vi "Multiply.vi"(8 "error in (no error)":errorcluster, 10 "Scale":dbl format="%#_13g", 11 "Field in":refnum<class "Field.lvclass">) -> (0 "error out":errorcluster, 3 "Field out":refnum<class "Field.lvclass">)   [LabVIEW 2020, in "Field.lvclass"]
uses:
  Field.lvclass
  Field.lvclass/Field.ctl
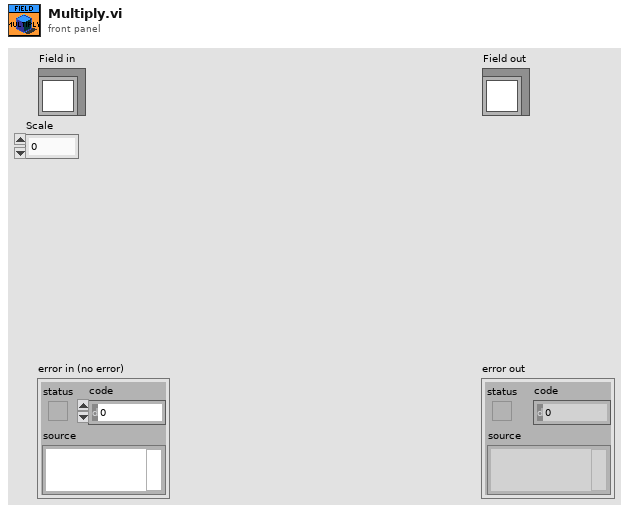
[diagram p1: front panel]
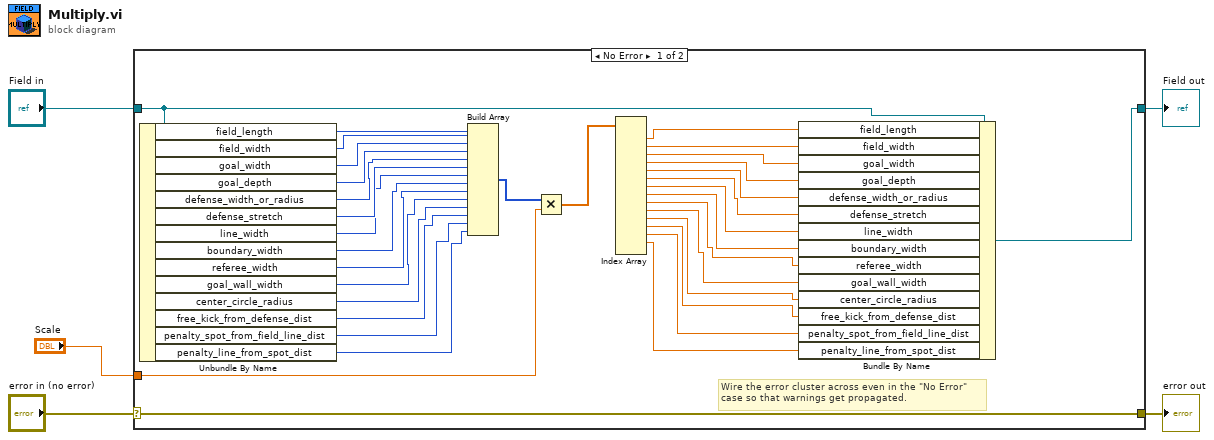
[diagram p0: block diagram]
diagram:
  n1 = case shown="No Error" "error in (no error)" {
    selector: "error in (no error)" -> [w39 w41]
    tunnel: [w39 w41] -> w4
    tunnel: [w37 w40] -> w2
    tunnel: "Field in" -> [w38 w40]
    tunnel: "Scale" -> [w30 _]
    frame No Error {
      # "Wire the error cluster across even in the \"No Error\"\ncase so that warnings get propagated."
      n2 = Unbundle By Name(w38) -> ("field_length"=w36:i32, "field_width"=w35:i32, "goal_width"=w34:i32, "goal_depth"=w33:i32, "defense_width_or_radius"=w32:i32, "defense_stretch"=w31:i32, "line_width"=w14:i32, "boundary_width"=w13:i32, "referee_width"=w12:i32, "goal_wall_width"=w11:i32, "center_circle_radius"=w10:i32, "free_kick_from_defense_dist"=w9:i32, "penalty_spot_from_field_line_dist"=w8:i32, "penalty_line_from_spot_dist"=w7:i32)
      n3 = Build Array(w36, w35, w34, w33, w32, w31, w14, w13, w12, w11, w10, w9, w8, w7) -> (w6:i32[])
      n4 = Multiply(x=w6, y=w30) -> (x*y=w29:dbl[])
      n5 = Index Array(array=w29) -> (element #1=w28:dbl, element #2=w27:dbl, element #3=w26:dbl, element #4=w25:dbl, element #5=w24:dbl, element #6=w23:dbl, element #7=w22:dbl, element #8=w21:dbl, element #9=w20:dbl, element #10=w19:dbl, element #11=w18:dbl, element #12=w17:dbl, element #13=w16:dbl, element #14=w15:dbl)  [unwired: 15 in, 1 out]
      n6 = Bundle By Name(cluster=w38, "field_length"=w28, "field_width"=w27, "goal_width"=w26, "goal_depth"=w25, "defense_width_or_radius"=w24, "defense_stretch"=w23, "line_width"=w22, "boundary_width"=w21, "referee_width"=w20, "goal_wall_width"=w19, "center_circle_radius"=w18, "free_kick_from_defense_dist"=w17, "penalty_spot_from_field_line_dist"=w16, "penalty_line_from_spot_dist"=w15) -> (w37:refnum<class "Field.lvclass">)
    }
    frame Error {
    }
  }
  "error out" <- w4
  "Field out" <- w2
